vi "init.vi"(8 "error in (no error)":errorcluster, 10 "WeatherData":refnum<class "WeatherData.lvclass">, 11 "CurrentConditionsDisplay in":refnum<class "CurrentConditionsDisplay.lvclass">) -> (0 "error out":errorcluster, 3 "CurrentConditionsDisplay out":refnum<class "CurrentConditionsDisplay.lvclass">)   [LabVIEW 2020, in "CurrentConditionsDisplay.lvclass"]
uses:
  CurrentConditionsDisplay.lvclass
  WeatherData/WeatherData.lvclass
  CurrentConditionsData.ctl
  CurrentConditionsDisplay.lvclass/CurrentConditionsDisplay.ctl
  DisplayBase/DisplayBase.lvclass
panel:
  # "Connector Pane"
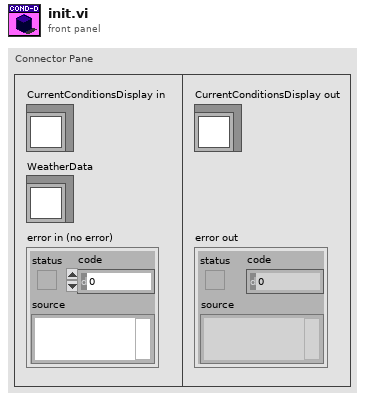
[diagram p1: front panel]
types:
  T1 = typedef "CurrentConditionsDisplay.lvclass/CurrentConditionsData.ctl" = cluster{"Temperature":dbl, "Humidity":dbl}
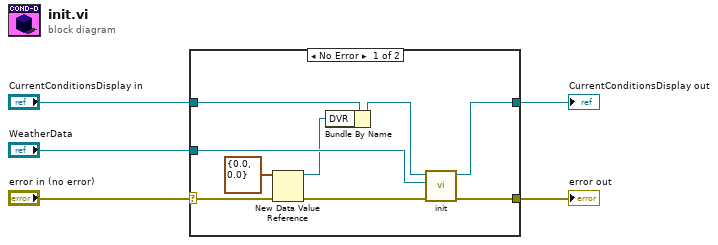
[diagram p0: block diagram]
diagram:
  n1 = case shown="No Error" "error in (no error)" {
    selector: "error in (no error)" -> [w10 w16]
    tunnel: [w14 w15] -> w5
    tunnel: "WeatherData" -> [w13 _]
    tunnel: "CurrentConditionsDisplay in" -> [w12 w15]
    tunnel: [w11 w16] -> w2
    frame No Error {
      n2 = New Data Value Reference(data value=T1 {"Temperature"=0.0, "Humidity"=0.0} ("CurrentConditionsData"), error in=w10) -> (data value reference=w6:refnum<data-value>, error out=w9:errorcluster)
      n3 = Bundle By Name(cluster=w12, "DVR"=w6) -> (w7:refnum<class "CurrentConditionsDisplay.lvclass">)
      n4 = call-parent "init.vi"("error in (no error)"=w9, "WeatherData"=w13, "DisplayBase in"=w7) -> ("error out"=w11:errorcluster, "DisplayBase out"=w14:refnum<class "CurrentConditionsDisplay.lvclass">)  [unwired: 7 in]
    }
    frame Error {
    }
  }
  "error out" <- w2
  "CurrentConditionsDisplay out" <- w5
